vi "GV FIFOINtimeout_tick.vi"() -> ()   [LabVIEW 2017]
panel:
  out "FIFOtimeout_tick":i32
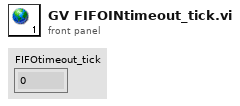
[diagram p1: front panel]
diagram:
